vi "Send Raw String.vi"(8 "error in (no error)":errorcluster, 10 "String Data":string, 11 "ENET in":refnum<class "ENET_BS120x.lvclass">) -> (0 "error out":errorcluster, 3 "ENET out":refnum<class "ENET_BS120x.lvclass">)   [LabVIEW 2021, in "BS120x Driver.lvlib" / "ENET_BS120x.lvclass"]
uses:
  ENET_BS120x.lvclass
  ENET_BS120x.lvclass/ENET_BS120x.ctl
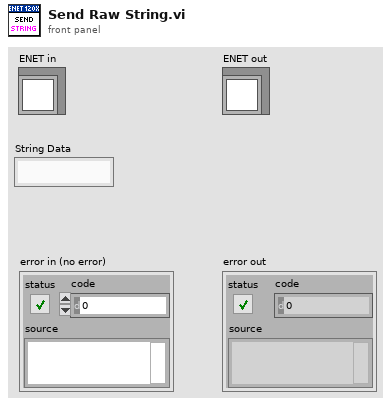
[diagram p1: front panel]
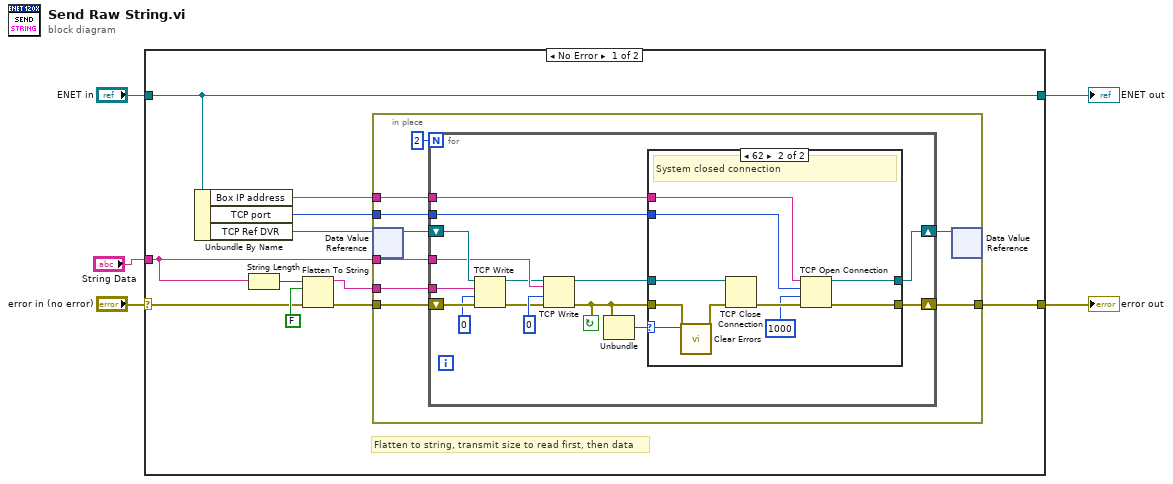
[diagram p0: block diagram]
diagram:
  n1 = case shown="No Error" "error in (no error)" {
    selector: "error in (no error)" -> [w7 w54]
    tunnel: [w10 w53] -> w5
    tunnel: "ENET in" -> [w10 w53]
    tunnel: [w12 w54] -> w3
    tunnel: "String Data" -> [w6 _]
    frame No Error {
      # "Flatten to string, transmit size to read first, then data"
      n2 = Unbundle By Name(w10) -> ("Box IP address"=w9:string, "TCP port"=w8:u16, "TCP Ref DVR"=w11:refnum<data-value>)
      n3 = String Length(string=w6) -> (length=w16:i32)
      n4 = Flatten To String(anything=w16, prepend array or string size? (T)=FALSE, error in (no error)=w7) -> (data string=w15:string, error out=w14:errorcluster)  [unwired: 1 in, 1 out]
      n5 = in-place {
        in-place-border: w15 -> [w25]
        in-place-border: w14 -> [w24]
        in-place-border: w6 -> [w23]
        in-place-border: [w22] -> w12
        in-place-border: w9 -> [w18]
        in-place-border: w8 -> [w17]
        n6 = in-place-dvr #1(w11) -> (w20:refnum<k5>)  [unwired: 1 out]
        n7 = for {
          N: 2 -> [_]
          tunnel: w25 -> [w38]
          tunnel: w23 -> [w34]
          shift-right: [w31] -> w19
          shift-left: w20 -> [w40]
          shift-right: [w29] -> w22
          shift-left: w24 -> [w37]
          tunnel: w18 -> [w27]
          tunnel: w17 -> [w26]
          stop <- w28 continue-if-true
          n8 = TCP Write(connection ID=w40, data in=w38, error in (no error)=w37, 9:0 ("timeout ms (25000)")) -> (connection ID out=w33:refnum<k5>, error out=w36:errorcluster)  [unwired: 1 out]
          n9 = TCP Write(connection ID=w33, data in=w34, error in (no error)=w36, 9:0 ("timeout ms (25000)")) -> (connection ID out=w32:refnum<k5>, error out=w28:errorcluster)  [unwired: 1 out]
          n10 = Unbundle(w28) -> ("code"=w30:i32)  [unwired: 2 out]
          n11 = case shown="62" w30 {
            selector: w30 -> [_ w45]
            tunnel: w32 -> [w42 w52]
            tunnel: [w41 w49] -> w29
            tunnel: [w42 w48] -> w31
            tunnel: w28 -> [w41 w51]
            tunnel: w27 -> [_ w44]
            tunnel: w26 -> [_ w43]
            frame 0, Default {
            }
            frame 62 {
              # "System closed connection"
              n12 = call <vilib>:"Clear Errors.vi"("error in (no error)"=w51, "specific error code to clear (0: all)"=w45) -> ("error out"=w46:errorcluster)  [unwired: 4 in, 1 out]
              n13 = TCP Close Connection(connection ID=w52, error in (no error)=w46) -> (error out=w50:errorcluster)  [unwired: 1 in, 1 out]
              n14 = TCP Open Connection(address=w44, remote port or service name=w43, timeout ms (60000)=1000 ("timeout ms (25000)"), error in (no error)=w50) -> (connection ID=w48:refnum<k5>, error out=w49:errorcluster)  [unwired: 1 in]
            }
          }
        }
        n15 = in-place-dvr #1(w19) -> ()  [unwired: 2 out]
      }
    }
    frame Error {
    }
  }
  "ENET out" <- w5
  "error out" <- w3
